vi "flinger_calc.vi"(11 "Flinger Inputs":T3) -> (3 "Flinger Outputs":T1)   [LabVIEW 2013]
uses:
  flinger_inputs.ctl
  flinger_outputs.ctl
  <vilib>/Rock Robotics/WPI/Solenoid/WPI_SolenoidValue.ctl
panel:
  in  "?":T1
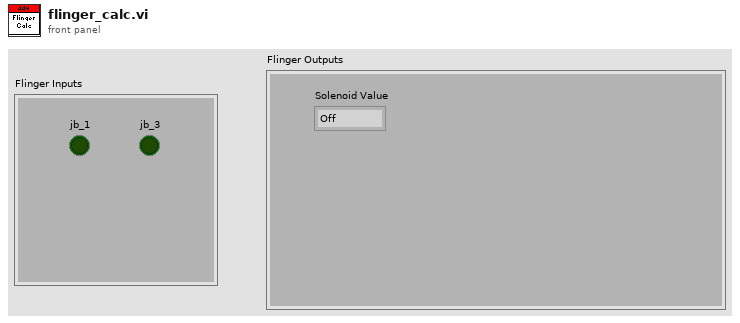
[diagram p1: front panel]
types:
  T1 = typedef "flinger_outputs.ctl" = cluster{"Solenoid Value":T2}
  T2 = typedef "WPI_SolenoidValue.ctl" = enum16{"Off", "On", "Forward", "Reverse"}
  T3 = typedef "flinger_inputs.ctl" = cluster{"jb_1":bool, "jb_3":bool}
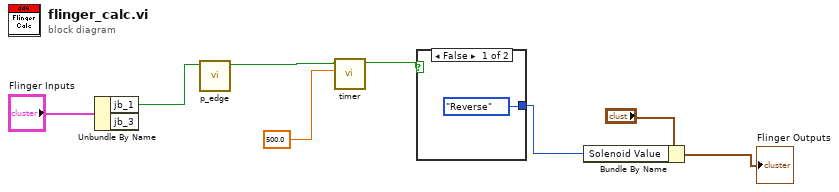
[diagram p0: block diagram]
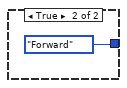
[diagram p2: hidden frame]
diagram:
  n1 = Unbundle By Name("Flinger Inputs") -> ("jb_1"=w7:bool)  [unwired: 1 out]
  n2 = call "p_edge.vi"("In"=w7) -> ("Out"=w5:bool)  [unwired: 10 in]
  n3 = call "timer.vi"("Time"=500.0, "Set"=w5) -> ("Out"=w6:bool)  [unwired: 9 in]
  n4 = case shown="False" w6 {
    tunnel: [WPI_SolenoidValue."Reverse" ("Solenoid 1 Value") WPI_SolenoidValue."Forward" ("Solenoid 1 Value")] -> w2
    frame False {
    }
    frame True {
    }
  }
  n5 = Bundle By Name(cluster="?", "Solenoid Value"=w2) -> (→"Flinger Outputs":T1)
